vi "Application name.vi"() -> (0 "Ini file path":path, 1 "download site":string, 2 "help site":string, 3 "application name":string)   [LabVIEW 2011, in "Design Server.lvlib"]
uses:
  Design Server.lvlib
panel:
  in  "default ini path for testing":path=path "C:/Users/design/Documents/Test.ini"
  out "Callers' Names":string[](array[string])
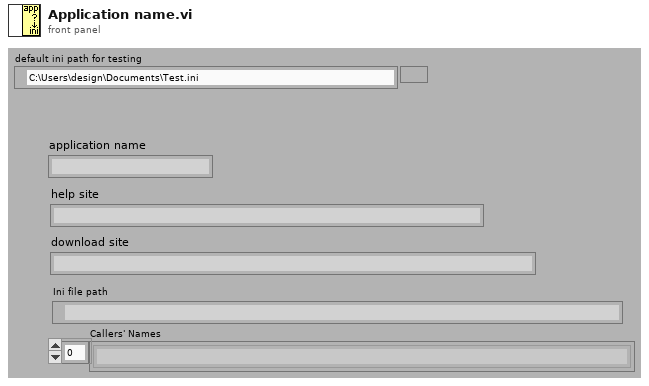
[diagram p1: front panel]
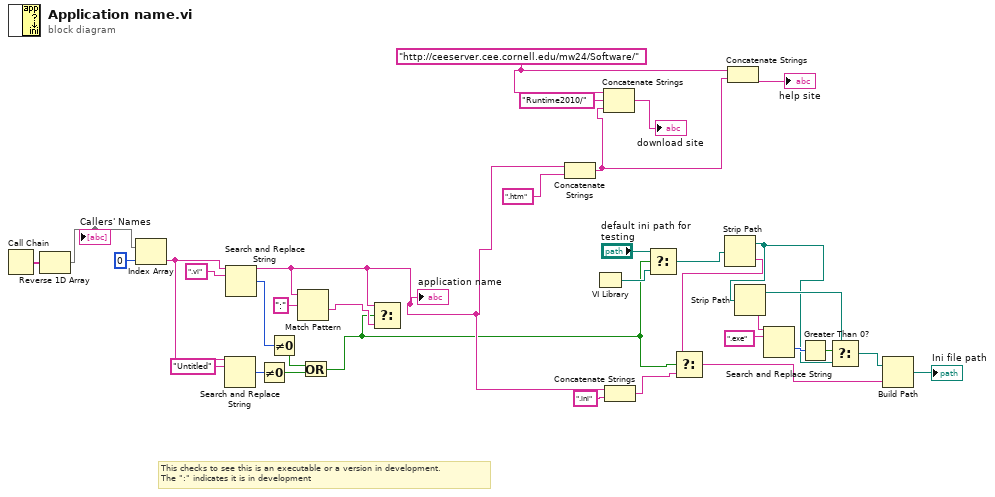
[diagram p0: block diagram]
diagram:
  w30 = "http://ceeserver.cee.cornell.edu/mw24/Software/"
  # "This checks to see this is an executable or a version in development.\nThe \":\" indicates it is in development"
  n1 = Call Chain() -> (call chain=w18:string[])
  n2 = Reverse 1D Array(array=w18) -> (reversed array=w17:string[])
  "Callers' Names" <- w17
  n3 = Index Array(array=w17, index=0) -> (element=w6:string)
  n4 = Search and Replace String(input string=w6, search string="Untitled") -> (number of replacements=w4:i32)  [unwired: 6 in, 3 out]
  n5 = Search and Replace String(input string=w6, search string=".vi" ("replace string (\"\")")) -> (result string=w12:string, number of replacements=w11:i32)  [unwired: 6 in, 2 out]
  "application name" <- w12
  n6 = Not Equal To 0?(x=w4) -> (x != 0?=w3:bool)
  n7 = Not Equal To 0?(x=w11) -> (x != 0?=w2:bool)
  n8 = Match Pattern(string=w12, regular expression=":") -> (after substring=w15:string)  [unwired: 1 in, 3 out]
  n9 = Or(x=w2, y=w3) -> (x .or. y?=w1:bool)
  n10 = Select(t=w12, s=w1, f=w15) -> ()  [unwired: 1 out]
  n11 = Concatenate Strings(w12, ".htm" ("replace string (\"\")")) -> (w28:string)
  n12 = VI Library() -> (path=w13:path)
  n13 = Concatenate Strings(w30, "Runtime2010/" ("string"), w28) -> (→"download site":string)
  n14 = Concatenate Strings(w12, ".ini") -> (w9:string)
  n15 = Select(t="default ini path for testing", s=w1, f=w13) -> (s? t:f=w14:path)
  n16 = Strip Path(path=w14) -> (stripped path=w22:path, name=w8:string)
  n17 = Select(t=w8, s=w1, f=w9) -> (s? t:f=w7:string)
  n18 = Concatenate Strings(w30, w28) -> (→"help site":string)
  n19 = Strip Path(path=w22) -> (stripped path=w23:path, name=w27:string)
  n20 = Search and Replace String(input string=w27, search string=".exe") -> (offset past replacement=w25:i32)  [unwired: 6 in, 3 out]
  n21 = Greater Than 0?(x=w25) -> (x > 0?=w24:bool)
  n22 = Select(t=w23, s=w24, f=w22) -> (s? t:f=w20:path)
  n23 = Build Path(base path=w20, name or relative path=w7) -> (appended path=→"Ini file path":path)
